vi "BenchmarkParams.vi"() -> (0 "error out":errorcluster, 3 "Numeric":dbl)   [LabVIEW 2011]
doc: "This code module is used for benchmarking the LabVIEW Adapter."
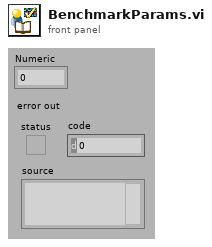
[diagram p1: front panel]
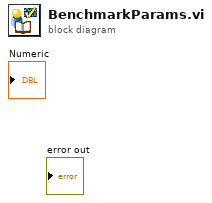
[diagram p0: block diagram]
diagram:
